vi "Test.vi"() -> ()   [LabVIEW 2014]
uses:
  spcm_library/spcm_gui_m4i.llb/element_device.ctl
  spcm_library/spcm_gui_m4i.llb/element_ao_channel.ctl
  spcm_library/spcm_gui_m4i.llb/element_ao_trigger.ctl
  spcm_library/spcm_gui_m4i.llb/element_mode_seq.ctl
  spcm_library/spcm_gui_m4i.llb/element_clock.ctl
  spcm_library/spcm_gui_m4i.llb/element_multi_purpose_io.ctl
  spcm_library/spcm_gui_m4i.llb/element_states_rep_seq.ctl
panel:
  in  "Multi Purpose IO Lines":T1={"X0 Mode"=0, "ASync Write"=8, "X1 Mode"=0, "X2 Mode"=0} {"X2 Mode" items=["Disable", "Asynchronous In", "Asynchronous Out", "Digital Input (A/D only)", "Digital Output (D/A only)", "Trigger Out", "Digital Input 2Bit (A/D only)", "Show Run State", "Show Arm State", "Ref Clock Out", "Output Marker (D/A only)", "System Clock Out"]; "X1 Mode" items=["Disable", "Asynchronous In", "Asynchronous Out", "Digital Input (A/D only)", "Digital Output (D/A only)", "Trigger Out", "Digital Input 2Bit (A/D only)", "Show Run State", "Show Arm State", "Ref Clock Out", "Output Marker (D/A only)", "System Clock Out"]; "ASync Write" min=8 step=4; "X0 Mode" items=["Disable", "Asynchronous In", "Asynchronous Out", "Digital Input (A/D only)", "Digital Output (D/A only)", "Trigger Out", "Digital Input 2Bit (A/D only)", "Show Run State", "Show Arm State", "Ref Clock Out", "Output Marker (D/A only)", "System Clock Out"]}
  in  "Clock Settings":T2={"Clock Mode"=1, "Sampling Rate (MHz)"=62.5, "Reference Clock (MHz)"=10.0, "Clock Output"=FALSE} {"Clock Mode" items=["Internal Clock Quartz", "External Clock (Reference Clock)"]; "Reference Clock (MHz)" min=10.0 max=125000.0; "Sampling Rate (MHz)" min=1.0 max=200000.0}
  in  "Sequence Step":T3 {"End condition" items=["End loop always", "End loop on trigger", "End sequence"]}
  in  "Sequence Steps":string[][](table)=[["0", "1", "0", "20000", "0"], ["1", "2", "1", "50000", "0"], ["2", "3", "0", "30000", "0"], ["3", "4", "2", "50000", "0"], ["4", "0", "0", "40000", "2"]]
  in  "Sequence Mode Setup":T4={"Number of segments"=4, "Start Segment"=0}
  out "Status":string="Stopped"
  in  "Trigger Settings":T5 {"Secondary Ext. Trigger" items=["None", "Pos. Edge", "Neg. Edge", "Any Edge", "High Level", "Low Level"]; "AC Coupling" items=["DC Coupling", "AC Coupling"]; "Main Ext. Trigger" items=["None", "Pos. Edge", "Neg. Edge", "Any Edge", "Pos. Rearm", "Neg. Rearm", "Enter Window", "Leave Window", "High Level", "Low Level", "In Win", "Out Win", ""]; "Trigger Source" items=["Software Trigger", "Main External Trigger", "Secondary External Trigger"]; "Trigger Delay (Samples)" max=65535 step=1}
  in  "Stop Level":cluster{"Stoplevel":u16}={"Stoplevel"=4} {"Stoplevel" items=["Tristate", "Low Level", "High Level", "Hold Last Sample", "Zero"]}
  in  "Output Channel 1":T6={"Enable"=TRUE, "Output Mode"=0, "Gain"=2000, "Offset"=0, "Filter"=0} {"Output Mode" items=["Single", "Double", "Differential"]}
  in  "Output Channel 0":T6={"Enable"=TRUE, "Output Mode"=0, "Gain"=2000, "Offset"=0, "Filter"=0} {"Output Mode" items=["Single", "Double", "Differential"]}
  in  "Singleshot Button":bool=TRUE
  out "Write Setup":bool
  in  "Quit Button":bool
  in  "Force Trigger Button":bool
  in  "Stop Button":bool
  out "Device Infos":T7={"Device Name"="M4i.6622-Exp", "Serial Number"=10722.0, "Mem (MB)"=4096.0}
  in  "Device":T8 {"Device" items=["Card", "digitizerNETBOX"]}
  # "Step"
  # "Next Step"
  # "Segment"
  # "Loops"
  # "End Condition*"
  # "Ch1"
  # "Ch0"
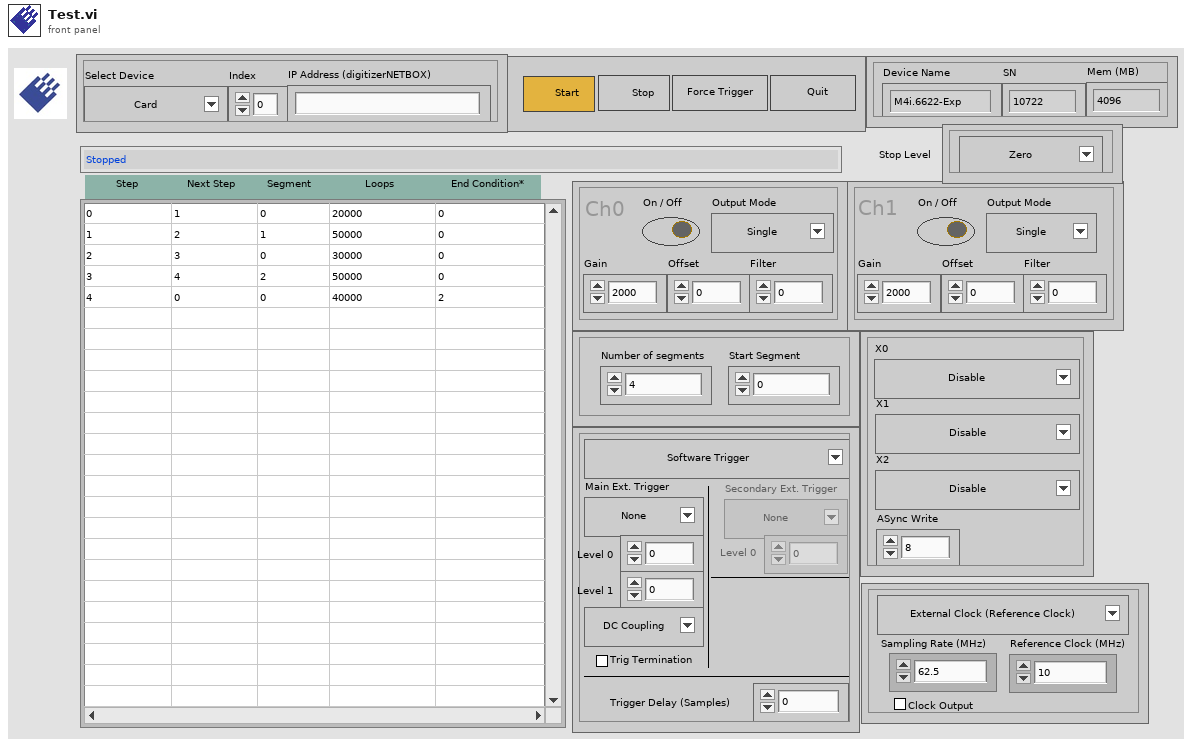
[diagram p1: front panel]
types:
  T1 = typedef "element_multi_purpose_io.ctl" = cluster{"X0 Mode":u16, "ASync Write":u32, "X1 Mode":u16, "X2 Mode":u16}
  T2 = typedef "element_clock.ctl" = cluster{"Clock Mode":u16, "Sampling Rate (MHz)":dbl, "Reference Clock (MHz)":dbl, "Clock Output":bool}
  T3 = cluster{"Step":i32, "Next Step":i32, "Segment":i32, "Loops":i32, "End condition":u16}
  T4 = typedef "element_mode_seq.ctl" = cluster{"Number of segments":u32, "Start Segment":u32}
  T5 = typedef "element_ao_trigger.ctl" = cluster{"Trigger Source":u16, "Main Ext. Trigger":u16, "Level 0 Ext":i32, "Level 1 Ext":i32, "AC Coupling":u16, "Ext Trig Term":bool, "Secondary Ext. Trigger":u16, "Level 0 Ext1":i32, "Trigger Delay (Samples)":u32}
  T6 = typedef "element_ao_channel.ctl" = cluster{"Enable":bool, "Output Mode":u16, "Gain":i32, "Offset":i32, "Filter":i32}
  T7 = cluster{"Device Name":string, "Serial Number":dbl, "Mem (MB)":dbl}
  T8 = typedef "element_device.ctl" = cluster{"Index":dbl, "IP Address":string, "Device":u16}
  T9 = typedef "element_states_rep_seq.ctl" = enum16{"Idle", "Init", "Write Setup", "Set Segment Data", "Set Segment Steps", "Start", "Replay", "Stop", "Quit"}
  T10 = cluster{"Card Type":i32, "Inst Mem (high part)":i32, "Serial Number":i32, "Function Type":i32, "Installed Features":i32, "Inst Mem (low part)":i32, "Base Card Version":i32, "Module Version":i32, "Extension Version":i32, "Production Date":i32, "Max Sampling Rate":i32, "Demo Card":i32}
  T11 = cluster{"Card Name":string, "SN":i32, "Mem (MB)":i32}
  T12 = cluster{"AO Channels":i32, "Bit Resolution":i32, "AO Gain":i32, "AO Filter":i32, "AO Offset":i32}
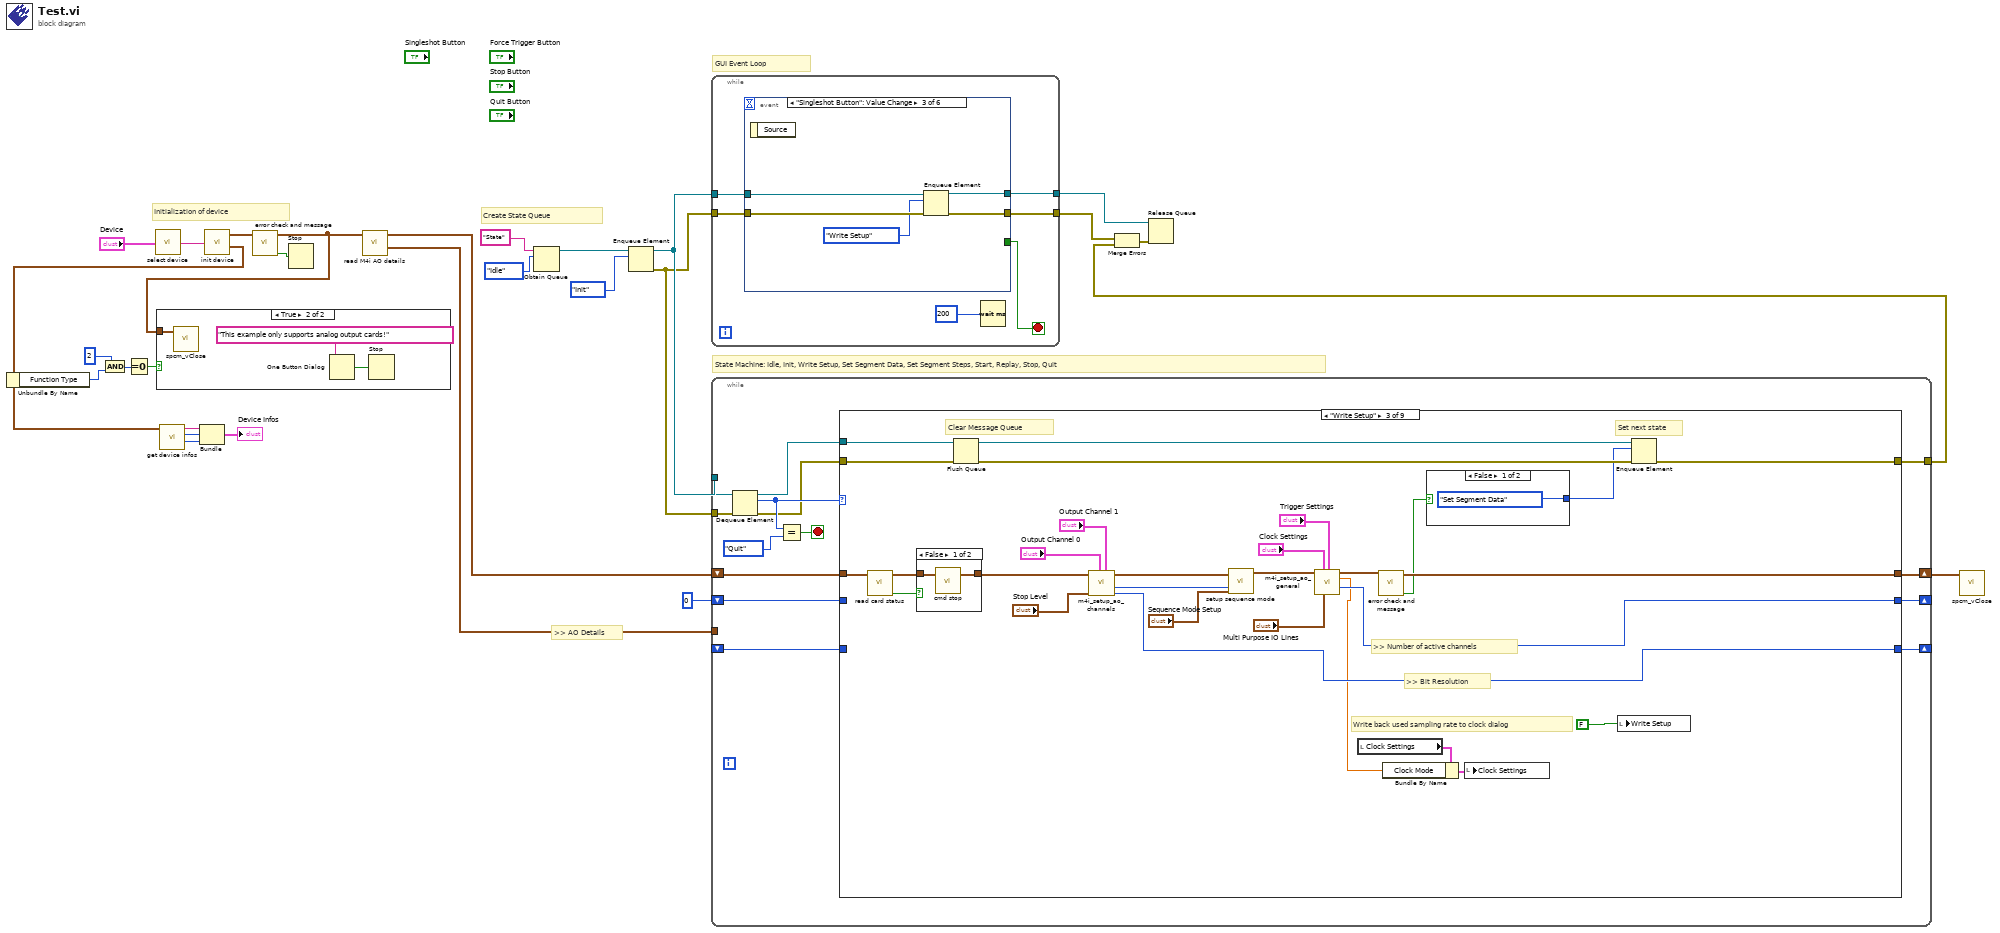
[diagram p0: block diagram]
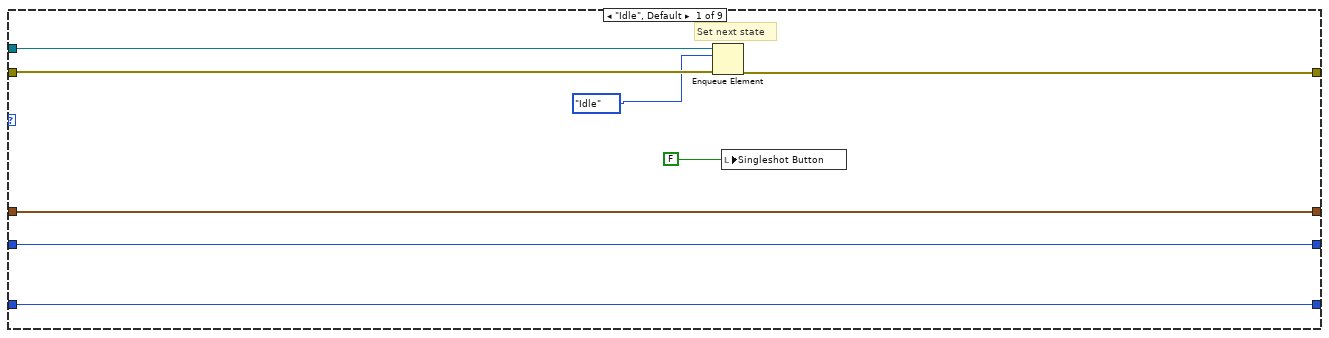
[diagram p3: hidden frame]
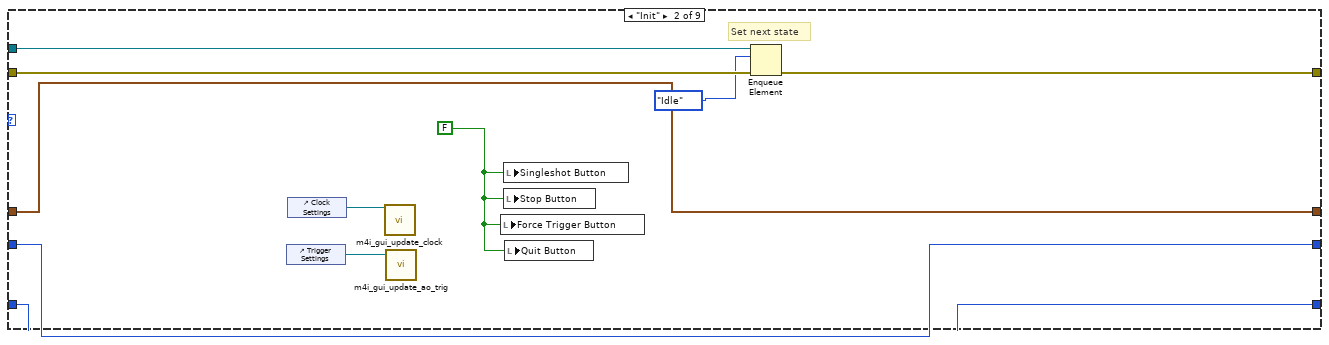
[diagram p4: hidden frame]
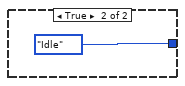
[diagram p6: hidden frame]
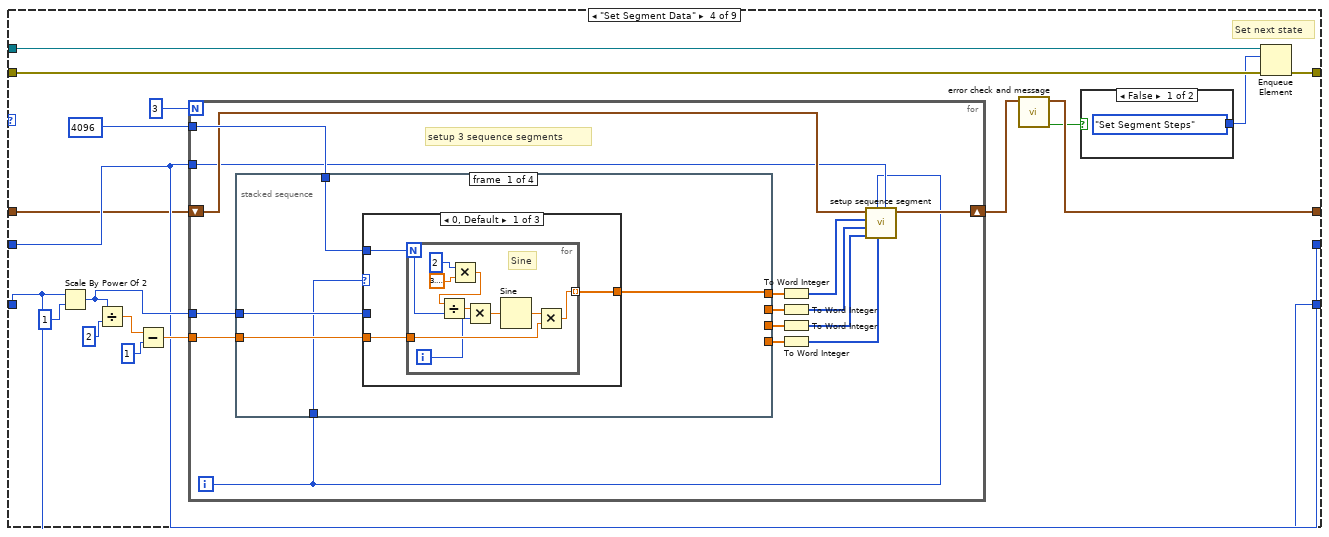
[diagram p7: hidden frame]
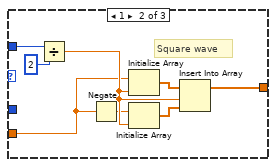
[diagram p8: hidden frame]
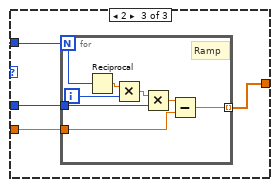
[diagram p9: hidden frame]
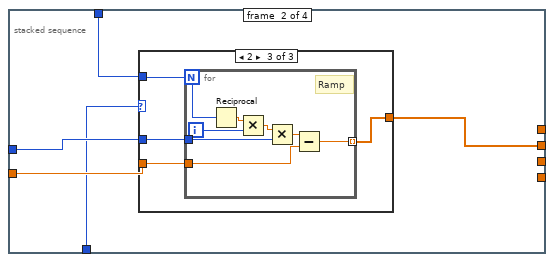
[diagram p10: hidden frame]
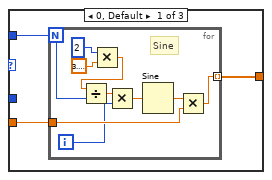
[diagram p11: hidden frame]
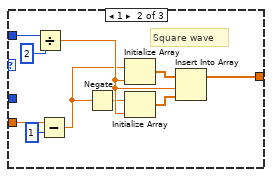
[diagram p12: hidden frame]
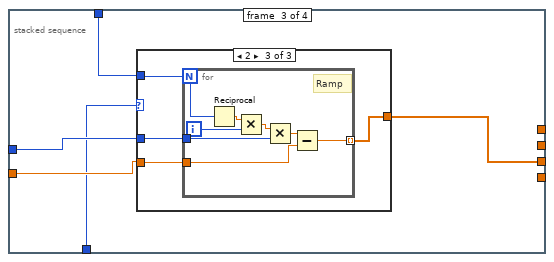
[diagram p13: hidden frame]
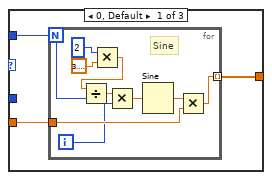
[diagram p14: hidden frame]
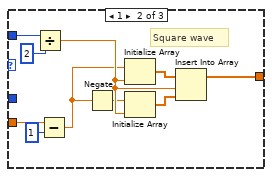
[diagram p15: hidden frame]
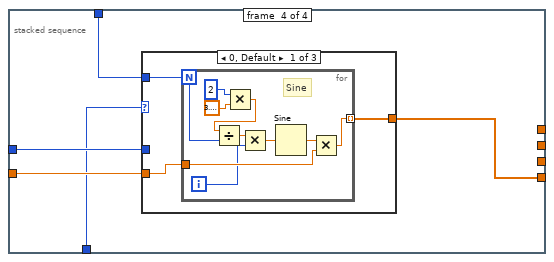
[diagram p16: hidden frame]
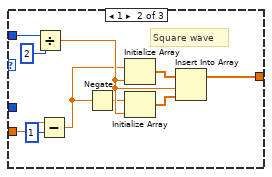
[diagram p17: hidden frame]
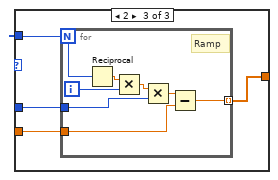
[diagram p18: hidden frame]
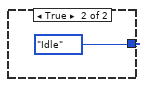
[diagram p19: hidden frame]
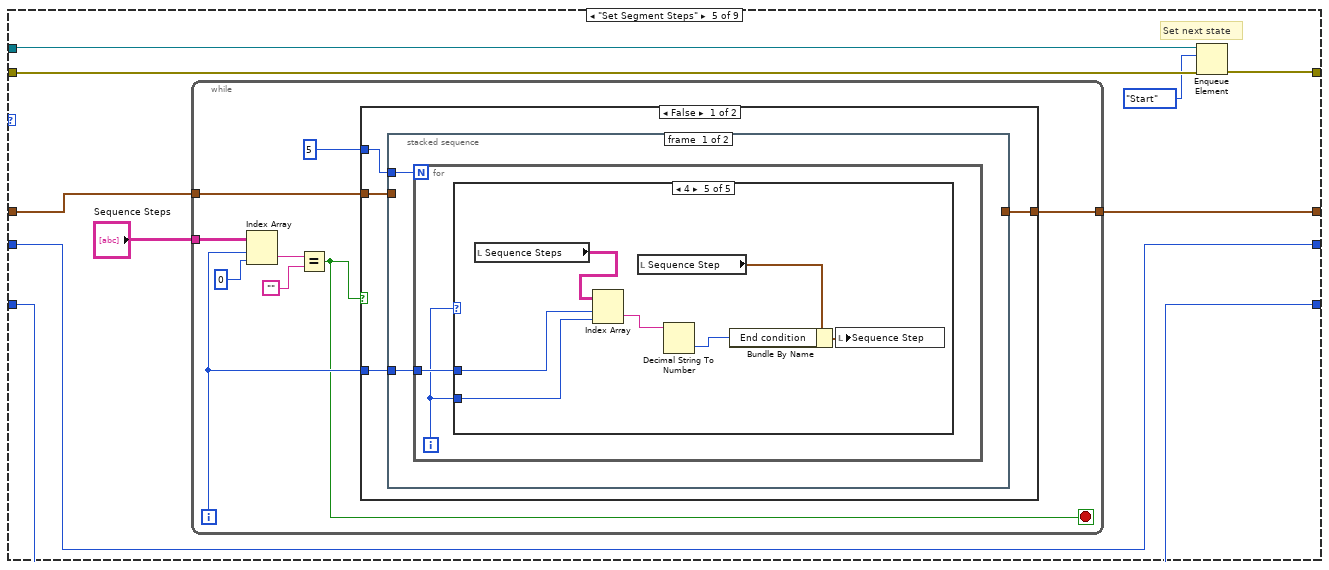
[diagram p20: hidden frame]
diagram:
  # ">> AO Details"
  # "Initialization of device"
  # "Create State Queue"
  # "State Machine: Idle, Init, Write Setup, Set Segment Data, Set Segment Steps, Start, Replay, Stop, Quit"
  # "GUI Event Loop"
  n1 = call "select device.vi"("Device"="Device") -> ("device string"=w28:string)  [unwired: 4 in]
  n2 = call "init device.vi"("Device String"=w28) -> ("Card Info Out"=w27:cluster{"Card Handle":u64, "Error Code":u32}, "Card Information"=w11:T10)  [unwired: 4 in]
  n3 = Unbundle By Name(w11) -> ("Function Type"=w15:i32)
  n4 = And(x=2, y=w15) -> (x .and. y?=w14:i32)
  n5 = Equal To 0?(x=w14) -> (x = 0?=w12:bool)
  n6 = call "get device infos.vi"("Card Information"=w11) -> ("Mem (MB)"=w19:i32, "SN"=w18:i32, "Card Name"=w17:string)  [unwired: 8 in]
  n7 = Bundle("Card Name"=w17, "SN"=w18, "Mem (MB)"=w19) -> (→"Device Infos":T11)  [unwired: 1 in]
  n8 = call "error check and message.vi"("Card Info In"=w27) -> ("Error occurred"=w26:bool, "Card Info Out"=w4:cluster{"Card Handle":u64, "Error Code":u32})  [unwired: 4 in, 1 out]
  n9 = case shown="True" w12 {
    tunnel: w4 -> [_ w29]
    frame False {
    }
    frame True {
      n10 = call "spcm_vClose.vi"("Card Info In"=w29) -> ()  [unwired: 7 in]
      n11 = One Button Dialog(message="This example only supports analog output cards!") -> (true=w30:bool)  [unwired: 1 in]
      n12 = Stop(stop? (T)=w30) -> ()
    }
  }
  n13 = Stop(stop? (T)=w26) -> ()
  n14 = call "read M4i AO details.vi"("Card Info In"=w4) -> ("AO Details"=w3:T12, "Card Info Out"=w2:cluster{"Card Handle":u64, "Error Code":u32})  [unwired: 5 in]
  n15 = Obtain Queue(name (unnamed)="State", element data type=element_states_rep_seq."Idle") -> (queue out=w23:refnum<queue>)  [unwired: 3 in, 2 out]
  n16 = Enqueue Element(queue=w23, element=element_states_rep_seq."Init") -> (queue out=w24:refnum<queue>, error out=w6:errorcluster)  [unwired: 2 in, 1 out]
  n17 = while {
    tunnel: w24 -> [w35]
    tunnel: [w36] -> w7
    tunnel: [w32] -> w10
    tunnel: w6 -> [w33]
    stop <- w34 stop-if-true
    n18 = event shown="[2] \"Singleshot Button\": Value Change" {
      selector: _ -> [_ _ _ _ _ _]
      dyn-events: _ -> [_ _ _ _ _ _]
      timeout: _ -> [_ _ _ _ _ _]
      tunnel: [_ _ _ _ TRUE _] -> w34
      tunnel: [w40 w43 w48 w53 w58 w62] -> w36
      tunnel: w35 -> [w40 w43 w47 w52 w59 w62]
      tunnel: [w39 w42 w45 w50 w56 w61] -> w32
      tunnel: w33 -> [w39 w42 w46 w51 w55 w61]
      event Value Change {
        n19 = event-data() -> ()  [unwired: 1 in, 1 out]
        n20 = control-ref of="Clock Settings"() -> (w38:refnum<vi>)
        n21 = call "m4i_gui_update_clock.vi"("Cluster Reference"=w38) -> ()  [unwired: 11 in]
      }
      event Value Change {
        n22 = event-data() -> ()  [unwired: 1 in, 1 out]
        n23 = control-ref of="Trigger Settings"() -> (w41:refnum<vi>)
        n24 = call "m4i_gui_update_ao_trig.vi"("Cluster Referenz"=w41) -> ()  [unwired: 11 in]
      }
      event "Singleshot Button": Value Change {
        n25 = event-data() -> ()  [unwired: 1 in, 1 out]
        n26 = Enqueue Element(queue=w47, element=element_states_rep_seq."Write Setup", error in (no error)=w46) -> (queue out=w48:refnum<queue>, error out=w45:errorcluster)  [unwired: 1 in, 1 out]
      }
      event "Stop Button": Value Change {
        n27 = event-data() -> ()  [unwired: 1 in, 1 out]
        n28 = Enqueue Element(queue=w52, element=element_states_rep_seq."Stop", error in (no error)=w51) -> (queue out=w53:refnum<queue>, error out=w50:errorcluster)  [unwired: 1 in, 1 out]
      }
      event "Quit Button": Value Change {
        n29 = event-data() -> ()  [unwired: 1 in, 1 out]
        n30 = Enqueue Element(queue=w59, element=element_states_rep_seq."Quit", error in (no error)=w55) -> (queue out=w58:refnum<queue>, error out=w56:errorcluster)  [unwired: 1 in, 1 out]
      }
      event Value Change {
        n31 = event-data() -> ()  [unwired: 1 in, 1 out]
        "Write Setup" <- TRUE
      }
    }
    n32 = Wait (ms)(milliseconds to wait=200) -> ()  [unwired: 1 out]
  }
  n33 = while {
    tunnel: w24 -> [w76]
    shift-right: [w74] -> w22
    shift-left: w2 -> [w75]
    shift-right: [w69] -> _
    shift-left: 0 -> [w70]
    tunnel: [w68] -> w9
    tunnel: w6 -> [w67]
    tunnel: w3 -> [_]
    shift-right: [w64] -> _
    shift-left: _ -> [w63]
    stop <- w72 stop-if-true
    n34 = Dequeue Element(queue=w76, error in (no error)=w67) -> (queue out=w71:refnum<queue>, element=w73:T9, error out=w66:errorcluster)  [unwired: 1 in, 1 out]
    n35 = Equal?(x=w73, y=element_states_rep_seq."Quit") -> (x = y?=w72:bool)
    n36 = case shown="\"Write Setup\"" w73 {
      tunnel: w75 -> [w84 w91 w107 w130 w328 w387 w406 w429 w436]
      tunnel: [w84 w91 w120 w134 w327 w386 w399 w428 w436] -> w74
      tunnel: w71 -> [w78 w94 w109 w144 w322 w393 w402 w432 _]
      tunnel: w70 -> [w83 w90 _ w136 w326 w392 w395 w427 w435]
      tunnel: [w83 w90 w116 w136 w326 w392 w395 w427 w435] -> w69
      tunnel: [w81 w93 w121 w143 w323 w391 w400 w430 w434] -> w68
      tunnel: w66 -> [w82 w92 w122 w145 w324 w390 _ w431 w434]
      tunnel: [w79 w86 w110 w135 w325 w388 w396 w425 w433] -> w64
      tunnel: w63 -> [w79 w86 _ w135 w325 w388 w396 w425 w433]
      frame "Idle", Default {
        # "Set next state"
        n37 = Enqueue Element(queue=w78, element=element_states_rep_seq."Idle", error in (no error)=w82) -> (error out=w81:errorcluster)  [unwired: 1 in, 2 out]
        n38 = local write "Singleshot Button"(FALSE) -> ()
      }
      frame "Init" {
        w89 = FALSE
        # "Set next state"
        n39 = control-ref of="Trigger Settings"() -> (w87:refnum<vi>)
        n40 = control-ref of="Clock Settings"() -> (w85:refnum<vi>)
        n41 = call "m4i_gui_update_clock.vi"("Cluster Reference"=w85) -> ()  [unwired: 11 in]
        n42 = call "m4i_gui_update_ao_trig.vi"("Cluster Referenz"=w87) -> ()  [unwired: 11 in]
        n43 = local write "Force Trigger Button"(w89) -> ()
        n44 = local write "Singleshot Button"(w89) -> ()
        n45 = local write "Stop Button"(w89) -> ()
        n46 = local write "Quit Button"(w89) -> ()
        n47 = Enqueue Element(queue=w94, element=element_states_rep_seq."Idle", error in (no error)=w92) -> (error out=w93:errorcluster)  [unwired: 1 in, 2 out]
      }
      frame "Write Setup" {
        # "Write back used sampling rate to clock dialog"
        # "Set next state"
        # "Clear Message Queue"
        # ">> Bit Resolution"
        # ">> Number of active channels"
        n48 = call "read card status.vi"("Card Info In"=w107) -> ("Card ready"=w104:bool, "Card Info Out"=w106:cluster{"Card Handle":u64, "Error Code":u32})  [unwired: 3 in, 2 out]
        n49 = case shown="False" w104 {
          tunnel: w106 -> [w124 w125]
          tunnel: [w123 w125] -> w105
          frame False {
            n50 = call "cmd stop.vi"("Card Info In"=w124) -> ("Card Info Out"=w123:cluster{"Card Handle":u64, "Error Code":u32})  [unwired: 6 in]
          }
          frame True {
          }
        }
        n51 = Flush Queue(queue=w109) -> (queue out=w108:refnum<queue>)  [unwired: 1 in, 2 out]
        n52 = call "m4i_setup_ao_channels.vi"("Output Channel 1"="Output Channel 1", "Output Channel 0"="Output Channel 0", "Stop Level"="Stop Level", "Card Info In"=w105) -> ("Bit Resolution"=w110:i32, "ChMask"=w101:i32, "Card Info Out"=w102:cluster{"Card Handle":u64, "Error Code":u32})  [unwired: 5 in]
        n53 = call "setup sequence mode.vi"("Sequence Mode Setup"="Sequence Mode Setup", "Channel  Mask Low"=w101, "Card Info In"=w102) -> ("Card Info Out"=w103:cluster{"Card Handle":u64, "Error Code":u32})  [unwired: 8 in]
        n54 = call "m4i_setup_ao_general.vi"("Card Info In"=w103, "Clock Settings"="Clock Settings", "Trigger Settings"="Trigger Settings", "Multi Purpose IO Lines"="Multi Purpose IO Lines") -> ("Card Info Out"=w111:cluster{"Card Handle":u64, "Error Code":u32}, "Used Sampling Rate (MS)"=w96:dbl, "Channel Count"=w116:i32)  [unwired: 7 in, 2 out]
        n55 = local read "Clock Settings"() -> (w98:T2)
        n56 = call "error check and message.vi"("Card Info In"=w111) -> ("Error occurred"=w119:bool, "Card Info Out"=w120:cluster{"Card Handle":u64, "Error Code":u32})  [unwired: 4 in, 1 out]
        n57 = Bundle By Name(cluster=w98, "Clock Mode"=w96) -> (w97:T2)
        n58 = case shown="False" w119 {
          tunnel: [element_states_rep_seq."Set Segment Data" element_states_rep_seq."Idle"] -> w118
          frame False {
          }
          frame True {
          }
        }
        n59 = local write "Clock Settings"(w97) -> ()
        n60 = local write "Write Setup"(FALSE) -> ()
        n61 = Enqueue Element(queue=w108, element=w118, error in (no error)=w122) -> (error out=w121:errorcluster)  [unwired: 1 in, 2 out]
      }
      frame "Set Segment Data" {
        # "Set next state"
        n62 = Scale By Power Of 2(n=w135, x=1) -> (x*2^n=w137:i32)
        n63 = Divide(x=w137, y=2) -> (x/y=w142:dbl)
        n64 = Subtract(x=w142, y=1) -> (x-y=w138:dbl)
        n65 = for {
          N: 3 ("y") -> [_]
          tunnel: w138 -> [w160]
          tunnel: w137 -> [w159]
          tunnel: w136 -> [w147]
          tunnel: 4096 ("y") -> [w154]
          shift-right: [w152] -> w128
          shift-left: w130 -> [w153]
          i -> [w146]
          # "setup 3 sequence segments"
          n66 = stacked-sequence {
            tunnel: [w162 _ _ _] -> w158
            tunnel: w154 -> [w165 w203 w243 w283]
            tunnel: [_ w200 _ _] -> w157
            tunnel: [_ _ w240 _] -> w156
            tunnel: [_ _ _ w280] -> w155
            tunnel: w160 -> [w164 w202 w242 w282]
            tunnel: w159 -> [w163 w201 w241 w281]
            tunnel: w146 -> [w161 w199 w239 w279]
            frame #0 {
              n67 = case shown="0, Default" w161 {
                tunnel: w165 -> [w168 w186 w190]
                tunnel: [w167 w182 w189] -> w162
                tunnel: w164 -> [w166 w179 w188]
                tunnel: w163 -> [_ _ w187]
                frame 0, Default {
                  n68 = for {
                    N: w168 -> [w171]
                    tunnel: [w169] -> w167 mode=indexing
                    tunnel: w166 -> [w177]
                    i -> [w172]
                    # "Sine"
                    n69 = Multiply(x=2, y=3.141592653589793) -> (x*y=w170:dbl)
                    n70 = Divide(x=w170, y=w171) -> (x/y=w173:dbl)
                    n71 = Multiply(x=w173, y=w172) -> (x*y=w174:dbl)
                    n72 = Sine(x=w174) -> (sin(x)=w178:dbl)
                    n73 = Multiply(x=w178, y=w177) -> (x*y=w169:dbl)
                  }
                }
                frame 1 {
                  # "Square wave"
                  n74 = Divide(x=w186, y=2) -> (x/y=w181:dbl)
                  n75 = Negate(x=w179) -> (-x=w180:dbl)
                  n76 = Initialize Array(w179, w181) -> (w184:dbl[])
                  n77 = Initialize Array(w180, w181) -> (w183:dbl[])
                  n78 = Insert Into Array(array=w184, index=w181, new element=w183) -> (w182:dbl[])
                }
                frame 2 {
                  n79 = for {
                    N: w190 -> [w193]
                    tunnel: [w195] -> w189 mode=indexing
                    tunnel: w188 -> [w192]
                    tunnel: w187 -> [w191]
                    i -> [w197]
                    # "Ramp"
                    n80 = Reciprocal(x=w193) -> (1/x=w198:dbl)
                    n81 = Multiply(x=w198, y=w197) -> (x*y=w196:dbl)
                    n82 = Multiply(x=w196, y=w191) -> (x*y=w194:dbl)
                    n83 = Subtract(x=w194, y=w192) -> (x-y=w195:dbl)
                  }
                }
              }
            }
            frame #1 {
              n84 = case shown="2" w199 {
                tunnel: w203 -> [w206 w226 w230]
                tunnel: [w205 w222 w229] -> w200
                tunnel: w202 -> [w204 w217 w228]
                tunnel: w201 -> [_ _ w227]
                frame 0, Default {
                  n85 = for {
                    N: w206 -> [w209]
                    tunnel: [w207] -> w205 mode=indexing
                    tunnel: w204 -> [w215]
                    i -> [w210]
                    # "Sine"
                    n86 = Multiply(x=2, y=3.141592653589793) -> (x*y=w208:dbl)
                    n87 = Divide(x=w208, y=w209) -> (x/y=w211:dbl)
                    n88 = Multiply(x=w211, y=w210) -> (x*y=w212:dbl)
                    n89 = Sine(x=w212) -> (sin(x)=w216:dbl)
                    n90 = Multiply(x=w216, y=w215) -> (x*y=w207:dbl)
                  }
                }
                frame 1 {
                  # "Square wave"
                  n91 = Divide(x=w226, y=2) -> (x/y=w221:dbl)
                  n92 = Subtract(x=w217, y=1) -> (x-y=w219:dbl)
                  n93 = Negate(x=w219) -> (-x=w220:dbl)
                  n94 = Initialize Array(w219, w221) -> (w224:dbl[])
                  n95 = Initialize Array(w220, w221) -> (w223:dbl[])
                  n96 = Insert Into Array(array=w224, index=w221, new element=w223) -> (w222:dbl[])
                }
                frame 2 {
                  n97 = for {
                    N: w230 -> [w233]
                    tunnel: [w235] -> w229 mode=indexing
                    tunnel: w228 -> [w232]
                    tunnel: w227 -> [w231]
                    i -> [w237]
                    # "Ramp"
                    n98 = Reciprocal(x=w233) -> (1/x=w238:dbl)
                    n99 = Multiply(x=w238, y=w237) -> (x*y=w236:dbl)
                    n100 = Multiply(x=w236, y=w231) -> (x*y=w234:dbl)
                    n101 = Subtract(x=w234, y=w232) -> (x-y=w235:dbl)
                  }
                }
              }
            }
            frame #2 {
              n102 = case shown="2" w239 {
                tunnel: w243 -> [w246 w266 w270]
                tunnel: [w245 w262 w269] -> w240
                tunnel: w242 -> [w244 w257 w268]
                tunnel: w241 -> [_ _ w267]
                frame 0, Default {
                  n103 = for {
                    N: w246 -> [w249]
                    tunnel: [w247] -> w245 mode=indexing
                    tunnel: w244 -> [w255]
                    i -> [w250]
                    # "Sine"
                    n104 = Multiply(x=2, y=3.141592653589793) -> (x*y=w248:dbl)
                    n105 = Divide(x=w248, y=w249) -> (x/y=w251:dbl)
                    n106 = Multiply(x=w251, y=w250) -> (x*y=w252:dbl)
                    n107 = Sine(x=w252) -> (sin(x)=w256:dbl)
                    n108 = Multiply(x=w256, y=w255) -> (x*y=w247:dbl)
                  }
                }
                frame 1 {
                  # "Square wave"
                  n109 = Divide(x=w266, y=2) -> (x/y=w261:dbl)
                  n110 = Subtract(x=w257, y=1) -> (x-y=w259:dbl)
                  n111 = Negate(x=w259) -> (-x=w260:dbl)
                  n112 = Initialize Array(w259, w261) -> (w264:dbl[])
                  n113 = Initialize Array(w260, w261) -> (w263:dbl[])
                  n114 = Insert Into Array(array=w264, index=w261, new element=w263) -> (w262:dbl[])
                }
                frame 2 {
                  n115 = for {
                    N: w270 -> [w273]
                    tunnel: [w275] -> w269 mode=indexing
                    tunnel: w268 -> [w272]
                    tunnel: w267 -> [w271]
                    i -> [w277]
                    # "Ramp"
                    n116 = Reciprocal(x=w273) -> (1/x=w278:dbl)
                    n117 = Multiply(x=w278, y=w277) -> (x*y=w276:dbl)
                    n118 = Multiply(x=w276, y=w271) -> (x*y=w274:dbl)
                    n119 = Subtract(x=w274, y=w272) -> (x-y=w275:dbl)
                  }
                }
              }
            }
            frame #3 {
              n120 = case shown="0, Default" w279 {
                tunnel: w283 -> [w286 w306 w310]
                tunnel: [w285 w302 w309] -> w280
                tunnel: w282 -> [w284 w297 w308]
                tunnel: w281 -> [_ _ w307]
                frame 0, Default {
                  n121 = for {
                    N: w286 -> [w289]
                    tunnel: [w287] -> w285 mode=indexing
                    tunnel: w284 -> [w295]
                    i -> [w290]
                    # "Sine"
                    n122 = Multiply(x=2, y=3.141592653589793) -> (x*y=w288:dbl)
                    n123 = Divide(x=w288, y=w289) -> (x/y=w291:dbl)
                    n124 = Multiply(x=w291, y=w290) -> (x*y=w292:dbl)
                    n125 = Sine(x=w292) -> (sin(x)=w296:dbl)
                    n126 = Multiply(x=w296, y=w295) -> (x*y=w287:dbl)
                  }
                }
                frame 1 {
                  # "Square wave"
                  n127 = Divide(x=w306, y=2) -> (x/y=w301:dbl)
                  n128 = Subtract(x=w297, y=1) -> (x-y=w299:dbl)
                  n129 = Negate(x=w299) -> (-x=w300:dbl)
                  n130 = Initialize Array(w299, w301) -> (w304:dbl[])
                  n131 = Initialize Array(w300, w301) -> (w303:dbl[])
                  n132 = Insert Into Array(array=w304, index=w301, new element=w303) -> (w302:dbl[])
                }
                frame 2 {
                  n133 = for {
                    N: w310 -> [w313]
                    tunnel: [w315] -> w309 mode=indexing
                    tunnel: w308 -> [w312]
                    tunnel: w307 -> [w311]
                    i -> [w317]
                    # "Ramp"
                    n134 = Reciprocal(x=w313) -> (1/x=w318:dbl)
                    n135 = Multiply(x=w318, y=w317) -> (x*y=w316:dbl)
                    n136 = Multiply(x=w316, y=w311) -> (x*y=w314:dbl)
                    n137 = Subtract(x=w314, y=w312) -> (x-y=w315:dbl)
                  }
                }
              }
            }
          }
          n138 = To Word Integer(number=w158) -> (16bit integer=w151:i16[])
          n139 = To Word Integer(number=w157) -> (16bit integer=w150:i16[])
          n140 = To Word Integer(number=w156) -> (16bit integer=w149:i16[])
          n141 = To Word Integer(number=w155) -> (16bit integer=w148:i16[])
          n142 = call "setup sequence segment.vi"("Number of channels"=w147, "Segment Data Ch3"=w148, "Segment number"=w146, "Segment Data Ch2"=w149, "Segment Data Ch1"=w150, "Segment Data Ch0"=w151, "Card Info In"=w153) -> ("Card Info Out"=w152:cluster{"Card Handle":u64, "Error Code":u32})  [unwired: 4 in]
        }
        n143 = call "error check and message.vi"("Card Info In"=w128) -> ("Error occurred"=w133:bool, "Card Info Out"=w134:cluster{"Card Handle":u64, "Error Code":u32})  [unwired: 4 in, 1 out]
        n144 = case shown="False" w133 {
          tunnel: [element_states_rep_seq."Set Segment Steps" element_states_rep_seq."Idle"] -> w132
          frame False {
          }
          frame True {
          }
        }
        n145 = Enqueue Element(queue=w144, element=w132, error in (no error)=w145) -> (error out=w143:errorcluster)  [unwired: 1 in, 2 out]
      }
      frame "Set Segment Steps" {
        # "Set next state"
        n146 = while {
          tunnel: "Sequence Steps" -> [w336]
          tunnel: w328 -> [w332]
          tunnel: [w331] -> w327
          i -> [w333]
          stop <- w330 stop-if-true
          n147 = Index Array(array=w336, index (row)=w333, index (col)=0) -> (element=w338:string)
          n148 = Equal?(x=w338, y="") -> (x = y?=w330:bool)
          n149 = case shown="False" w330 {
            tunnel: 5 -> [w342 _]
            tunnel: w333 -> [w341 _]
            tunnel: w332 -> [w340 w385]
            tunnel: [w339 w385] -> w331
            frame False {
              n150 = stacked-sequence {
                tunnel: w342 -> [w344 _]
                tunnel: w341 -> [w343 _]
                tunnel: w340 -> [_ w384]
                tunnel: [_ w383] -> w339
                frame #0 {
                  n151 = for {
                    N: w344 -> [_]
                    tunnel: w343 -> [w346]
                    i -> [w345]
                    n152 = case shown="4" w345 {
                      tunnel: w346 -> [w347 w354 w361 w368 w375]
                      tunnel: w345 -> [w348 w358 w365 w372 w379]
                      frame 0, Default {
                        n153 = local read "Sequence Steps"() -> (w350:string[][])
                        n154 = Index Array(array=w350, index (row)=w347, index (col)=w348) -> (element=w349:string)
                        n155 = local read "Sequence Step"() -> (w352:T3)
                        n156 = Decimal String To Number(string=w349) -> (number=w353:i32)  [unwired: 2 in, 1 out]
                        n157 = Bundle By Name(cluster=w352, "Step"=w353) -> (w351:T3)
                        n158 = local write "Sequence Step"(w351) -> ()
                      }
                      frame 1 {
                        n159 = local read "Sequence Steps"() -> (w360:string[][])
                        n160 = Index Array(array=w360, index (row)=w354, index (col)=w358) -> (element=w359:string)
                        n161 = Decimal String To Number(string=w359) -> (number=w357:i32)  [unwired: 2 in, 1 out]
                        n162 = local read "Sequence Step"() -> (w355:T3)
                        n163 = Bundle By Name(cluster=w355, "Next Step"=w357) -> (w356:T3)
                        n164 = local write "Sequence Step"(w356) -> ()
                      }
                      frame 2 {
                        n165 = local read "Sequence Steps"() -> (w367:string[][])
                        n166 = Index Array(array=w367, index (row)=w361, index (col)=w365) -> (element=w366:string)
                        n167 = local read "Sequence Step"() -> (w362:T3)
                        n168 = Decimal String To Number(string=w366) -> (number=w364:i32)  [unwired: 2 in, 1 out]
                        n169 = Bundle By Name(cluster=w362, "Segment"=w364) -> (w363:T3)
                        n170 = local write "Sequence Step"(w363) -> ()
                      }
                      frame 3 {
                        n171 = local read "Sequence Steps"() -> (w374:string[][])
                        n172 = Index Array(array=w374, index (row)=w368, index (col)=w372) -> (element=w373:string)
                        n173 = local read "Sequence Step"() -> (w369:T3)
                        n174 = Decimal String To Number(string=w373) -> (number=w371:i32)  [unwired: 2 in, 1 out]
                        n175 = Bundle By Name(cluster=w369, "Loops"=w371) -> (w370:T3)
                        n176 = local write "Sequence Step"(w370) -> ()
                      }
                      frame 4 {
                        n177 = local read "Sequence Steps"() -> (w381:string[][])
                        n178 = Index Array(array=w381, index (row)=w375, index (col)=w379) -> (element=w380:string)
                        n179 = local read "Sequence Step"() -> (w377:T3)
                        n180 = Decimal String To Number(string=w380) -> (number=w376:i32)  [unwired: 2 in, 1 out]
                        n181 = Bundle By Name(cluster=w377, "End condition"=w376) -> (w378:T3)
                        n182 = local write "Sequence Step"(w378) -> ()
                      }
                    }
                  }
                }
                frame #1 {
                  # "write sequence step"
                  n183 = call "setup sequence step.vi"("Sequence Step"="Sequence Step", "Card Info In"=w384) -> ("Card Info Out"=w383:cluster{"Card Handle":u64, "Error Code":u32})  [unwired: 9 in]
                }
              }
            }
            frame True {
            }
          }
        }
        n184 = Enqueue Element(queue=w322, element=element_states_rep_seq."Start", error in (no error)=w324) -> (error out=w323:errorcluster)  [unwired: 1 in, 2 out]
      }
      frame "Start" {
        # "Set next state"
        n185 = call "cmd start.vi"("Card Info In"=w387) -> ("Card Info Out"=w386:cluster{"Card Handle":u64, "Error Code":u32})  [unwired: 6 in]
        n186 = Enqueue Element(queue=w393, element=element_states_rep_seq."Replay", error in (no error)=w390) -> (error out=w391:errorcluster)  [unwired: 1 in, 2 out]
      }
      frame "Replay" {
        # "Set next state"
        n187 = call "read card status.vi"("Card Info In"=w406) -> ("Card ready"=w398:bool, "Trigger detected"=w408:bool, "Pretrigger full"=w407:bool, "Card Info Out"=w405:cluster{"Card Handle":u64, "Error Code":u32})  [unwired: 3 in]
        n188 = call "spcm_translate_status_out.vi"("Ready"=w398, "Trigger"=w408, "Pretrigger"=w407) -> ("Text"=→"Status":string)  [unwired: 4 in]
        n189 = call "error check and message.vi"("Card Info In"=w405) -> ("Error occurred"=w404:bool)  [unwired: 4 in, 2 out]
        n190 = Not(x=w404) -> (.not. x?=w403:bool)
        n191 = case shown="True" w403 {
          tunnel: [element_states_rep_seq."Quit" w414] -> w401
          tunnel: w398 -> [_ w419]
          frame False {
          }
          frame True {
            n192 = local read "Write Setup"() -> (w413:bool)
            n193 = local read "Stop Button"() -> (w416:bool)
            n194 = Select(t=element_states_rep_seq."Idle", s=w419, f=element_states_rep_seq."Replay") -> (s? t:f=w411:T9)
            n195 = Select(t=element_states_rep_seq."Write Setup", s=w413, f=w411) -> (s? t:f=w410:T9)
            n196 = Select(t=element_states_rep_seq."Stop", s=w416, f=w410) -> (s? t:f=w414:T9)
          }
        }
        n197 = local read "Force Trigger Button"() -> (w394:bool)
        n198 = Enqueue Element(queue=w402, element=w401) -> (error out=w400:errorcluster)  [unwired: 2 in, 2 out]
        n199 = case shown="True" w394 {
          tunnel: w405 -> [w420 w421]
          tunnel: [w420 w423] -> w399
          frame False {
          }
          frame True {
            n200 = local write "Force Trigger Button"(FALSE) -> ()
            n201 = call "cmd force trigger.vi"("Card Info In"=w421) -> ("Card Info Out"=w423:cluster{"Card Handle":u64, "Error Code":u32})  [unwired: 6 in]
          }
        }
      }
      frame "Stop" {
        # "Set next state"
        n202 = call "cmd stop.vi"("Card Info In"=w429) -> ("Card Info Out"=w428:cluster{"Card Handle":u64, "Error Code":u32})  [unwired: 6 in]
        n203 = Enqueue Element(queue=w432, element=element_states_rep_seq."Idle", error in (no error)=w431) -> (error out=w430:errorcluster)  [unwired: 1 in, 2 out]
        n204 = local write "Status"("Stopped") -> ()
      }
      frame "Quit" {
      }
    }
  }
  n205 = Merge Errors(w10, w9) -> (w8:errorcluster)
  n206 = Release Queue(queue=w7, error in (no error)=w8) -> ()  [unwired: 1 in, 3 out]
  n207 = call "spcm_vClose.vi"("Card Info In"=w22) -> ()  [unwired: 7 in]
